vi "EnqueLowPriority.vi"(8 "error in (no error)":errorcluster, 10 "message":variant, 11 "queue in":refnum<data-value>) -> (0 "error out":errorcluster, 3 "queue out":refnum<data-value>)   [LabVIEW 2009, in "PriorityQueue.lvlib"]
uses:
  PriorityQueue.lvlib
  PriorityQueue/PriorityQueue.lvclass
  LLNode/LLNode.lvclass
  LowPriority/LowPriority.lvclass
  LinkedList/position.ctl
  LinkedList/LinkedList.lvclass
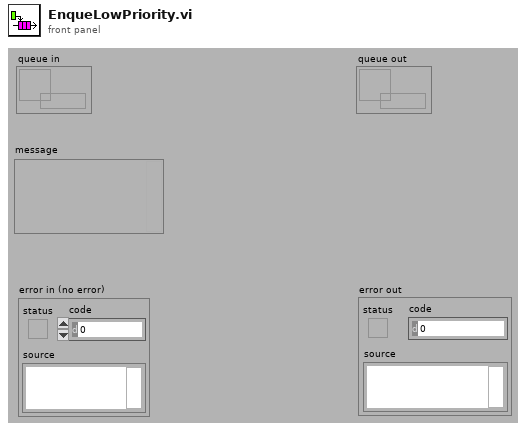
[diagram p1: front panel]
types:
  T1 = typedef "LinkedList.lvclass/position.ctl" = enum16{"Front", "Back", "Search"}
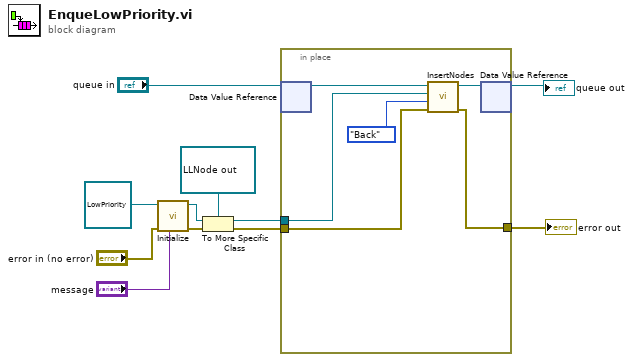
[diagram p0: block diagram]
diagram:
  n1 = call-dynamic "Initialize.vi"("optional"="message", "error in (no error)"="error in (no error)", "LowPriority data"=refnum<class "LowPriority.lvclass"> refnum ("LowPriority.lvclass")) -> ("error out"=w9:errorcluster, "Node out"=w8:refnum<data-value>)  [unwired: 7 in]
  n2 = To More Specific Class(target class=refnum<data-value> refnum ("ToInsert"), reference=w8, error in=w9) -> (specific class reference=w6:refnum<data-value>, error out=w1:errorcluster)
  n3 = in-place {
    in-place-border: w6 -> [w14]
    in-place-border: w1 -> [w15]
    in-place-border: [w12] -> w4
    n4 = in-place-dvr #1("queue in") -> (w17:refnum<class "PriorityQueue.lvclass">)  [unwired: 1 out]
    n5 = call "InsertNodes.vi"("error in (no error)"=w15, "position"=position."Back", "ToInsert"=w14, "LinkedList in"=w17) -> ("error out"=w12:errorcluster, "LinkedList out"=w13:refnum<class "PriorityQueue.lvclass">)  [unwired: 5 in, 1 out]
    n6 = in-place-dvr #1(w13) -> (→"queue out":refnum<data-value>)  [unwired: 1 out]
  }
  "error out" <- w4
